vi "Check Nodes.vi"(8 "error in (no error)":errorcluster, 11 "TelemetryDebug in":refnum<class "TelemetryDebug.lvclass">) -> (0 "error out":errorcluster, 3 "TelemetryDebug out":refnum<class "TelemetryDebug.lvclass">)   [LabVIEW 2020, in "VectoTools.lvlib" / "TelemetryDebug.lvclass"]
uses:
  TelemetryDebug.lvclass
  TelemetryDebug.lvclass/TelemetryDebug.ctl
  <vilib>/Utility/miscctls.llb/LVMapReplaceAction.ctl
  Vecto/NodeDiscovery/NodeDiscovery.lvclass
  Vecto/RemoteDataService/RemoteDataService.lvclass
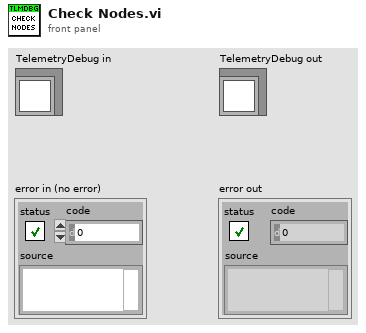
[diagram p1: front panel]
types:
  T1 = typedef "Discovery.lvlib/Data.ctl" = cluster{"node_id":u32, "name":string, "ip":u32, "status":string, "services":T2[], "system":string, "cluster":string, "app_version":string, "cfg_version":string}
  T2 = typedef "Service.lvlib/Data.ctl" = cluster{"type":T3, "port":i32}
  T3 = typedef "ServiceType.lvlib/Enumeration.ctl" = enum16{"SERVICETYPE_UNKNOWN", "SERVICETYPE_TCPSERVER", "SERVICETYPE_HTTPSERVER"}
  T4 = typedef "LVMapReplaceAction.ctl" = enum32{"Modify Entry only if found", "Add or Modify Entry", "Delete Entry"}
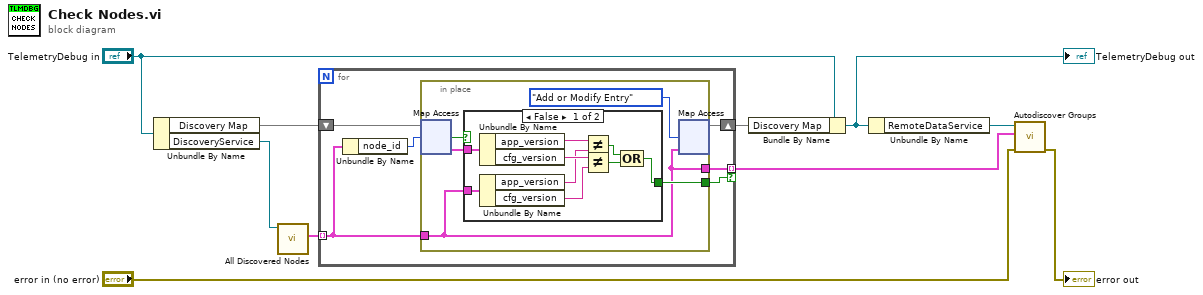
[diagram p0: block diagram]
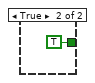
[diagram p2: hidden frame]
diagram:
  n1 = Unbundle By Name("TelemetryDebug in") -> ("Discovery Map"=w8:map{u32, T1}, "DiscoveryService"=w10:refnum<class "NodeDiscovery.lvclass">)
  n2 = call "All Discovered Nodes.vi"("DiscoveryService in"=w10) -> ("Nodes"=w9:T1[])  [unwired: 8 in, 2 out]
  n3 = for {
    tunnel: w9 -> [w14] mode=indexing
    shift-right: [w13] -> w7
    shift-left: w8 -> [w16]
    tunnel: [w12] -> w3 mode=indexing if=w11
    n4 = Unbundle By Name(w14) -> ("node_id"=w15:u32)
    n5 = in-place {
      in-place-border: w14 -> [w17]
      in-place-border: [w17] -> w12
      in-place-border: [w18] -> w11
      n6 = in-place-map #1(w16, w15) -> (w20:T1, w21:bool)  [unwired: 1 in]
      n7 = case shown="False" w21 {
        tunnel: w20 -> [w30 _]
        tunnel: [w22 TRUE] -> w18
        tunnel: w17 -> [w29 _]
        frame False {
          n8 = Unbundle By Name(w30) -> ("app_version"=w27:string, "cfg_version"=w28:string)
          n9 = Unbundle By Name(w29) -> ("app_version"=w26:string, "cfg_version"=w25:string)
          n10 = Not Equal?(x=w27, y=w26) -> (x != y?=w23:bool)
          n11 = Not Equal?(x=w28, y=w25) -> (x != y?=w24:bool)
          n12 = Compound Arithmetic op=OR(w23, w24) -> (w22:bool)
        }
        frame True {
        }
      }
      n13 = in-place-map #1(w17, LVMapReplaceAction."Add or Modify Entry" ("action")) -> (w13:map{u32, T1})  [unwired: 2 out]
    }
  }
  n14 = Bundle By Name(cluster="TelemetryDebug in", "Discovery Map"=w7) -> (w5:refnum<class "TelemetryDebug.lvclass">)
  "TelemetryDebug out" <- w5
  n15 = Unbundle By Name(w5) -> ("RemoteDataService"=w4:refnum<class "RemoteDataService.lvclass">)
  n16 = call "Autodiscover Groups.vi"("error in (no error)"="error in (no error)", "Groups"=w3, "RemoteDataService in"=w4) -> ("error out"=→"error out":errorcluster)  [unwired: 7 in, 1 out]
